vi "9871 EPICS - FPGA - Decode Received FIFO U16.vi"(11 "U16":u16 format="%016b") -> (1 "Parameter High Nibble Mid 4 bits  (xxNNNNxx xxxxxxxx)":u8 format="%04b", 2 "Low Byte (xxxxxxxx NNNNNNNN)":u8 format="%.0x", 3 "Request Type":T1(ring), 5 "Port# (1-4)":u8, 7 "Port Bits Only in U16":u16 format="%016b")   [LabVIEW 2020]
panel:
  out "2nd Nibble Low 2 bits  (xxxxxxNN xxxxxxxx)":u8 format="%02b"
  out "2nd Nibble HIgh 2 bits  (xxxxNNxx xxxxxxxx)":u8 format="%02b"
  out "High Byte (NNNNNNNN xxxxxxxx) Bin":u8 format="%08b"
  out "High Byte (NNNNNNNN xxxxxxxx) Hex":u8 format="%.0x"
  out "High Nibble (NNNNxxxx xxxxxxxx)":u8 format="%.0x"
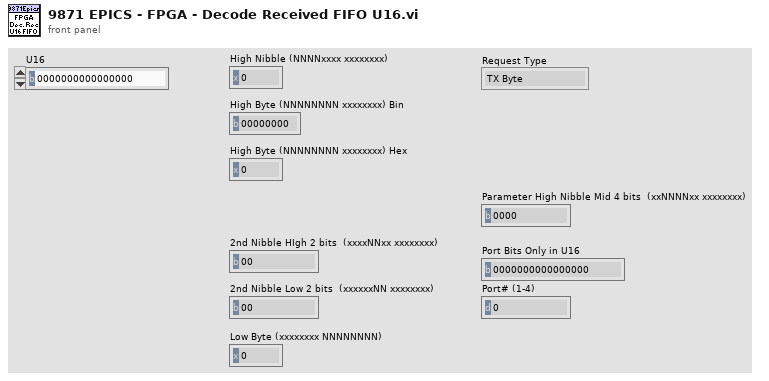
[diagram p1: front panel]
types:
  T1 = enum16{"TX Byte", "TX Clear", "Echo Request", "Parameter Change"}
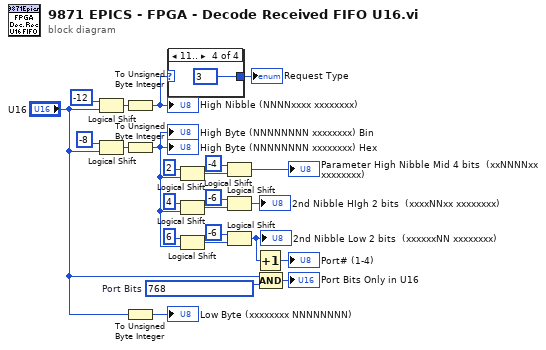
[diagram p0: block diagram]
diagram:
  w5 = u16 768  # Port Bits
  n1 = Logical Shift(y=i16 -12, x="U16") -> (x << y=w23:u16)
  n2 = Logical Shift(y=i16 -8, x="U16") -> (x << y=w22:u16)
  n3 = To Unsigned Byte Integer(number=w23) -> (unsigned 8bit integer=w1:u8)
  "High Nibble (NNNNxxxx xxxxxxxx)" <- w1
  n4 = To Unsigned Byte Integer(number=w22) -> (unsigned 8bit integer=w3:u8)
  "High Byte (NNNNNNNN xxxxxxxx) Hex" <- w3
  "High Byte (NNNNNNNN xxxxxxxx) Bin" <- w3
  n5 = To Unsigned Byte Integer(number="U16") -> (unsigned 8bit integer=→"Low Byte (xxxxxxxx NNNNNNNN)":u8)
  n6 = case shown="11.." w1 {
    selector: w1 -> [w25 w26 w27 _]
    tunnel: [w25 w26 w27 u8 3] -> w11
    frame 0 {
    }
    frame 1 {
    }
    frame 2 {
    }
    frame 3.. {
    }
  }
  "Request Type" <- w11
  n7 = Logical Shift(y=i16 2, x=w3) -> (x << y=w17:u8)
  n8 = Logical Shift(y=i16 4, x=w3) -> (x << y=w14:u8)
  n9 = Logical Shift(y=i16 6, x=w3) -> (x << y=w8:u8)
  n10 = Logical Shift(y=i16 -4, x=w17) -> (x << y=→"Parameter High Nibble Mid 4 bits  (xxNNNNxx xxxxxxxx)":u8)
  n11 = Logical Shift(y=i16 -6, x=w14) -> (x << y=→"2nd Nibble HIgh 2 bits  (xxxxNNxx xxxxxxxx)":u8)
  n12 = Logical Shift(y=i16 -6, x=w8) -> (x << y=w2:u8)
  "2nd Nibble Low 2 bits  (xxxxxxNN xxxxxxxx)" <- w2
  n13 = Increment(x=w2) -> (x+1=→"Port# (1-4)":u8)
  n14 = Compound Arithmetic op=AND("U16", w5) -> (→"Port Bits Only in U16":u16)
